vi "Start.vi"(8 "error in (no error)":errorcluster, 10 "Message in":refnum<class "StartMessage.lvclass">, 11 "AOTF in":refnum<class "Invivo_AOTF.lvclass">) -> (0 "error out":errorcluster, 3 "AOTF out":refnum<class "Invivo_AOTF.lvclass">)   [LabVIEW 2012, in "Invivo_AOTF.lvclass"]
doc: "This member function is called when the statemachine in the run.vi receives an 'start' command. It relays the message to all observers of the component.\n\nOverride this member function in your derived class if you need additional start functionality (but don't forget to call the parent method)."
uses:
  Invivo_AOTF.lvclass
  <vilib>/Distrio/Murmex/StartMessage/StartMessage.lvclass
  <vilib>/Distrio/Murmex/Murmex/Murmex.lvclass
panel:
  # "This member function is called when the statemachine in the run.vi receives an 'start' command. It relays the message to all observers of the component.\n\nOverride this member function in your derived class if you need additional start functionality (but don't forget to call the parent method)."
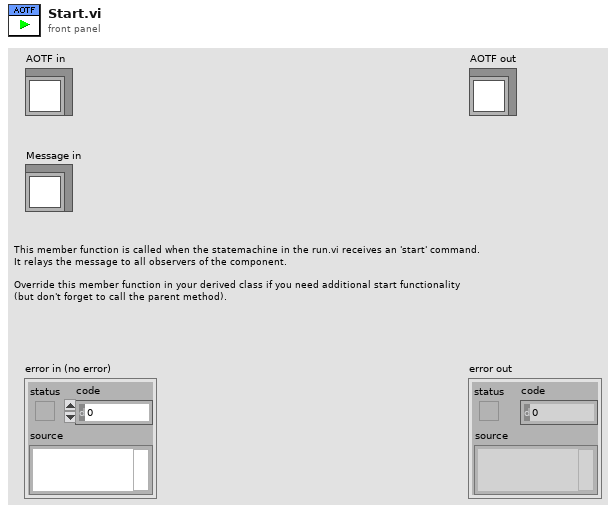
[diagram p1: front panel]
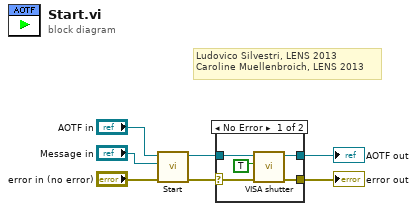
[diagram p0: block diagram]
diagram:
  # "Ludovico Silvestri, LENS 2013\nCaroline Muellenbroich, LENS 2013"
  n1 = call-parent "Start.vi"("error in (no error)"="error in (no error)", "Message in"="Message in", "Murmex in"="AOTF in") -> ("error out"=w2:errorcluster, "Murmex out"=w1:refnum<class "Invivo_AOTF.lvclass">)  [unwired: 7 in]
  n2 = case shown="No Error" w2 {
    selector: w2 -> [w12 w13]
    tunnel: [w8 w13] -> w7
    tunnel: [w9 w14] -> w6
    tunnel: w1 -> [w11 w14]
    frame No Error {
      n3 = call-dynamic "VISA shutter.vi"("error in (no error)"=w12, "button::shutter"=TRUE, "AOTF in"=w11) -> ("error out"=w8:errorcluster, "AOTF out"=w9:refnum<class "Invivo_AOTF.lvclass">)  [unwired: 7 in]
    }
    frame Error {
    }
  }
  "error out" <- w7
  "AOTF out" <- w6
